vi "Main - Process - Protected.vi"(8 "error in (no error)":errorcluster) -> (0 "error out":errorcluster)   [LabVIEW 2011]
doc: "This is a basic Queue Driven Message Handler VI. Most advanced LabVIEW programmers who code extensively in LabVIEW utilitze some variation of this VI. This is a starting point. Some key features need to be added. In particular a robust error handling routine should be added.\n\nAAL 9/09"
uses:
  Shared/QDMH Poly VIs/QDMH POLY Enqueue Strings.vi
  Shared/QDMH Poly VIs/QDMH POLY Enqueue String.vi
panel:
  out "Recent Cases":string
  out "Message Display":string
  in  "Cancel":bool
  in  "OK":bool
  # "Run this VI and run Main - Interrupt Process.vi.  When you press the Interrupt Process button, the interruption is controlled and only happens between Process 3 and Process 1.  Notice how the messages are queued at the same time in the Timeout case in this VI.\nAlso, consider writting a more intelligent block of code to intercept the messages coming in."
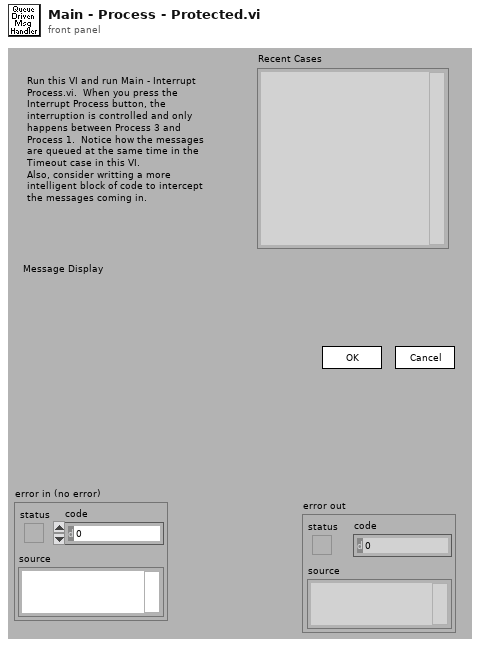
[diagram p1: front panel]
types:
  T1 = cluster{"Operator Name":string, "Current VI's Path":path, "Current VI's  Directory":path, "Queue Names":string[], "# VIs Launched":i32}
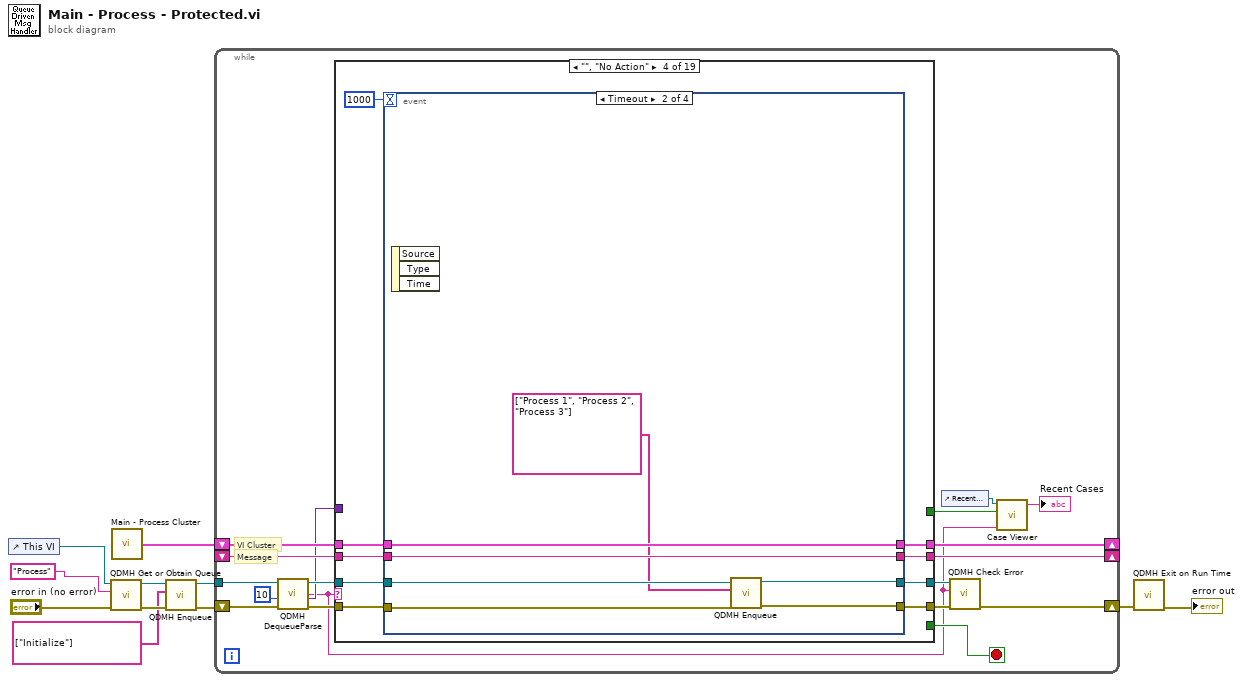
[diagram p0: block diagram]
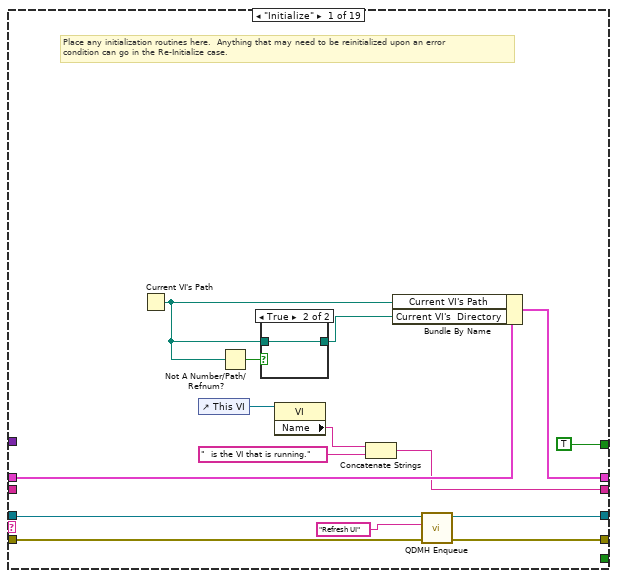
[diagram p2: hidden frame]
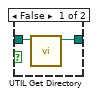
[diagram p3: hidden frame]
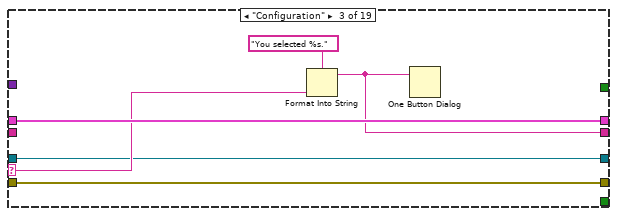
[diagram p5: hidden frame]
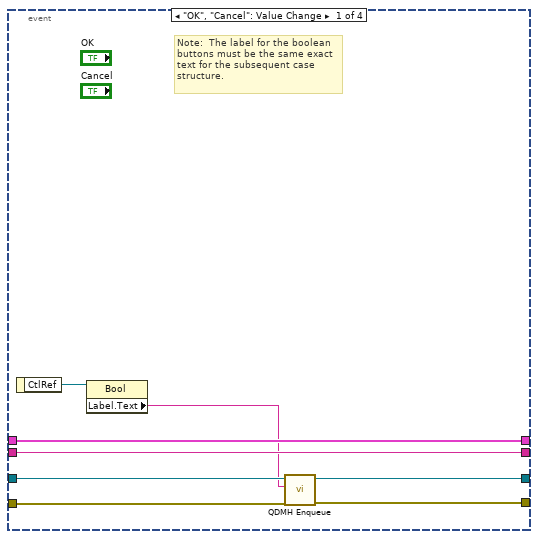
[diagram p6: hidden frame]
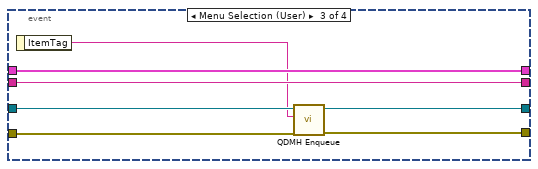
[diagram p7: hidden frame]
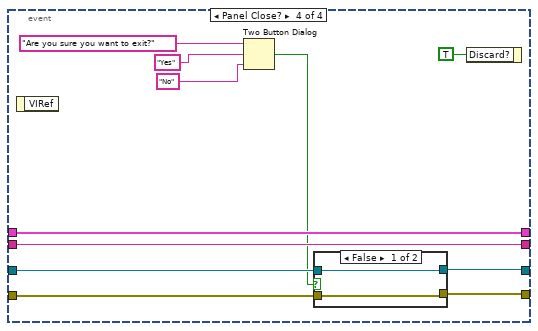
[diagram p8: hidden frame]
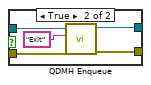
[diagram p9: hidden frame]
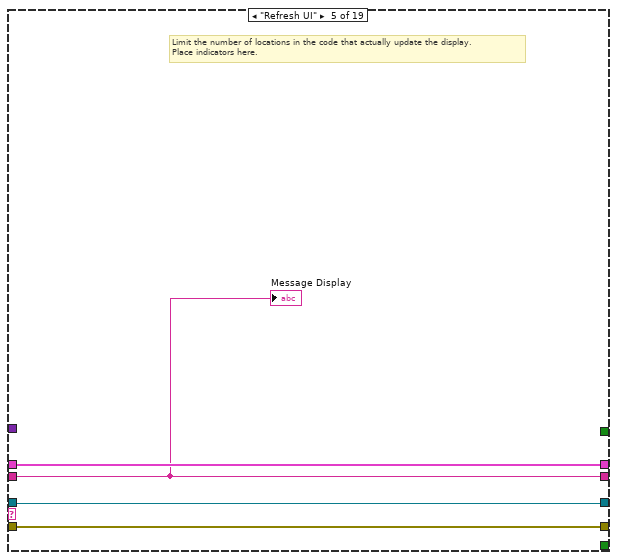
[diagram p10: hidden frame]
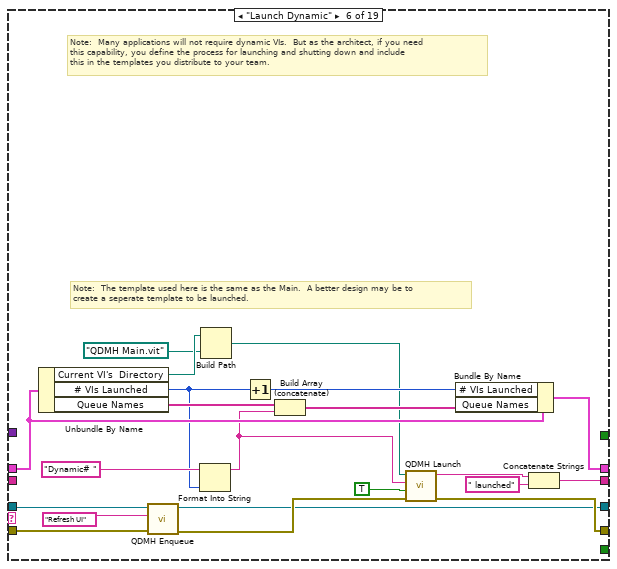
[diagram p11: hidden frame]
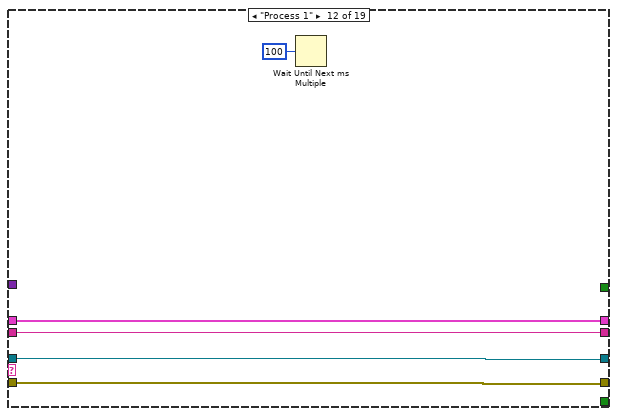
[diagram p17: hidden frame]
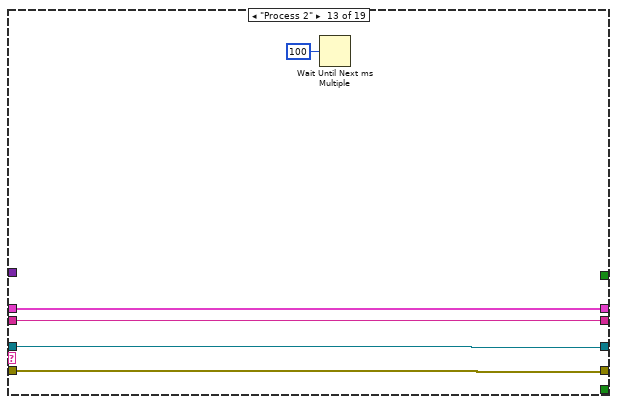
[diagram p18: hidden frame]
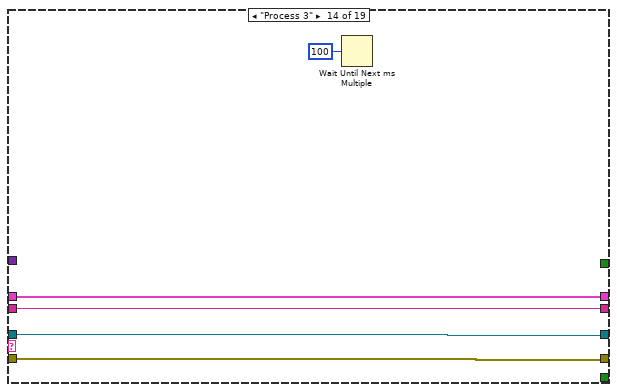
[diagram p19: hidden frame]
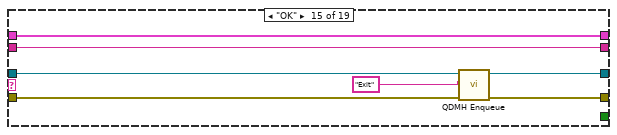
[diagram p20: hidden frame]
diagram:
  n1 = control-ref of="This VI"() -> (w5:refnum<vi>)
  n2 = call "QDMH Get or Obtain Queue.vi"("error in (no error)"="error in (no error)", "Queue Name"="Process", "VI Refnum"=w5) -> ("error out"=w8:errorcluster, "queue out"=w9:refnum<queue>)  [unwired: 7 out]
  n3 = call "Main - Process Cluster.vi"() -> ("Cluster"=w11:T1)
  n4 = call-poly "QDMH Enqueue.vi"("error in (no error)"=w8, "States"=string[] ["Initialize"], "queue"=w9) -> ("error out"=w6:errorcluster, "queue out"=w7:refnum<queue>)  [unwired: 7 out]
  n5 = while {
    tunnel: w7 -> [w24]
    shift-left: w11 -> [w25]
    shift-right: [w26] -> _
    shift-left: _ -> [w27]
    shift-right: [w28] -> _
    shift-right: [w18] -> w4
    shift-left: w6 -> [w20]
    stop <- w29 stop-if-true
    # "VI Cluster"
    # "Message"
    n6 = call "QDMH DequeueParse.vi"("error in (no error)"=w20, "Timeout"=10 ("ms timeout (-1)"), "queue"=w24) -> ("error out"=w21:errorcluster, "Variant Data"=w16:variant, "State"=w12:string, "queue out"=w22:refnum<queue>)  [unwired: 5 out]
    n7 = case shown="\"\", \"No Action\"" w12 {
      selector: w12 -> [_ _ w54 _ _ _ _ _ _ _ _ _ _ _ _ _ _ w193 _]
      tunnel: w22 -> [w40 w48 w53 w66 w108 w127 w132 w136 w140 w144 w148 w154 w159 w164 w173 w175 w187 w190 w203]
      tunnel: [_ _ _ _ _ _ _ _ _ _ _ _ _ _ _ _ _ _ TRUE] -> w29
      tunnel: [w38 w51 w55 w59 w109 w128 w135 w139 w143 w147 w151 w156 w161 w166 w172 w177 w189 w196 w205] -> w28
      tunnel: w27 -> [_ w51 _ w60 w109 _ w135 w139 w143 w147 w151 w156 w161 w166 w172 w177 w189 w196 w205]
      tunnel: [w43 w50 w57 w61 w110 w124 w134 w138 w142 w146 w150 w155 w160 w165 w171 w176 w188 w195 w200] -> w26
      tunnel: w25 -> [w44 w50 w57 w62 w110 w125 w134 w138 w142 w146 w150 w155 w160 w165 w171 w176 w188 w195 w200]
      tunnel: w21 -> [w42 w49 w52 w65 w107 w118 w133 w137 w141 w145 w149 w153 w158 w163 w170 w174 _ w192 w202]
      tunnel: [w41 w49 w52 w64 w107 w117 w133 w137 w141 w145 w149 w153 w158 w163 w169 w174 w186 w192 w197] -> w19
      tunnel: [w33 w48 w53 w58 w108 w114 w132 w136 w140 w144 w148 w154 w159 w164 w167 w175 w185 w190 refnum<queue> refnum ("queue out")] -> w17
      tunnel: w16 -> [_ _ _ _ _ _ _ _ _ _ _ _ _ _ _ _ w183 _ _]
      tunnel: [TRUE _ _ _ _ _ _ _ _ _ _ _ _ _ _ _ _ _ _] -> w14
      frame "Initialize" {
        # "Place any initialization routines here.  Anything that may need to be reinitialized upon an error\ncondition can go in the Re-Initialize case."
        n8 = Current VI's Path() -> (path=w31:path)
        n9 = control-ref of="This VI"() -> (w37:refnum<vi>)
        n10 = Not A Number/Path/Refnum?(number/path/refnum=w31) -> (NaN/Path/Refnum?=w32:bool)
        n11 = case shown="True" w32 {
          tunnel: w31 -> [w46 w47]
          tunnel: [w45 w47] -> w35
          frame False {
            n12 = call "UTIL Get Directory.vi"("Path In"=w46) -> ("Directory Out"=w45:path)  [unwired: 1 in, 9 out]
          }
          frame True {
          }
        }
        n13 = property class="VI"(reference=w37) -> ("Name"=w36:string)  [unwired: 1 in, 2 out]
        n14 = Concatenate Strings(w36, "  is the VI that is running." ("string")) -> (w38:string)
        n15 = Bundle By Name(cluster=w44, "Current VI's Path"=w31, "Current VI's  Directory"=w35) -> (w43:T1)
        n16 = call-poly "QDMH Enqueue.vi"("error in (no error)"=w42, "State"="Refresh UI" ("New State"), "queue"=w40) -> ("error out"=w41:errorcluster, "queue out"=w33:refnum<queue>)  [unwired: 7 out]
      }
      frame "Re-Initialize" {
        # "This case includes initialization functionality that may need to run again during the course of the VI"
      }
      frame "Configuration" {
        n17 = Format Into String(format string="You selected %s." ("Format String"), w54) -> (resulting string=w55:string)  [unwired: 2 in, 1 out]
        n18 = One Button Dialog(message=w55) -> ()  [unwired: 2 out]
      }
      frame "", "No Action" {
        n19 = event shown="[1] Timeout" {
          selector: _ -> [_ _ _ _]
          dyn-events: _ -> [_ _ _ _]
          timeout: 1000 -> [_ _ _ _]
          tunnel: w66 -> [w73 w79 w88 w95]
          tunnel: [w72 w76 w86 w92] -> w64
          tunnel: w65 -> [w71 w78 w87 w94]
          tunnel: w62 -> [w70 w81 w85 w99]
          tunnel: [w70 w81 w85 w99] -> w61
          tunnel: w60 -> [w69 w80 w84 w98]
          tunnel: [w69 w80 w84 w98] -> w59
          tunnel: [w67 w77 w82 w93] -> w58
          event "OK", "Cancel": Value Change {
            # "Note:  The label for the boolean buttons must be the same exact text for the subsequent case structure."
            n20 = event-data() -> ("CtlRef"=w74:refnum<vi>)  [unwired: 1 out]
            n21 = property class="Bool"(reference=w74) -> ("Label.Text"=w68:string)  [unwired: 1 in, 2 out]
            n22 = call-poly "QDMH Enqueue.vi"("error in (no error)"=w71, "State"=w68, "queue"=w73) -> ("error out"=w72:errorcluster, "queue out"=w67:refnum<queue>)  [unwired: 7 out]
          }
          event Timeout {
            n23 = event-data() -> ()  [unwired: 4 out]
            n24 = call-poly "QDMH Enqueue.vi"("error in (no error)"=w78, "States"=string[] ["Process 1", "Process 2", "Process 3"], "queue"=w79) -> ("error out"=w76:errorcluster, "queue out"=w77:refnum<queue>)  [unwired: 7 out]
          }
          event Menu Selection (User) {
            n25 = event-data() -> ("ItemTag"=w83:string)  [unwired: 1 out]
            n26 = call-poly "QDMH Enqueue.vi"("error in (no error)"=w87, "State"=w83, "queue"=w88) -> ("error out"=w86:errorcluster, "queue out"=w82:refnum<queue>)  [unwired: 7 out]
          }
          event Panel Close? {
            n27 = event-data() -> ()  [unwired: 2 out]
            n28 = Two Button Dialog(message="Are you sure you want to exit?", 1:"No" ("T button name (\"OK\")"), 2:"Yes" ("F button name (\"Cancel\")")) -> (T button?=w89:bool)
            n29 = case shown="False" w89 {
              tunnel: w95 -> [w101 w106]
              tunnel: w94 -> [w100 w105]
              tunnel: [w101 w104] -> w93
              tunnel: [w100 w103] -> w92
              frame False {
              }
              frame True {
                n30 = call-poly "QDMH Enqueue.vi"("error in (no error)"=w105, "State"="Exit", "queue"=w106) -> ("error out"=w103:errorcluster, "queue out"=w104:refnum<queue>)  [unwired: 7 out]
              }
            }
            n31 = event-data("Discard?"=TRUE) -> ()  [unwired: 1 in, 1 out]
          }
        }
      }
      frame "Refresh UI" {
        # "Limit the number of locations in the code that actually update the display.\nPlace indicators here."
        "Message Display" <- w109
      }
      frame "Launch Dynamic" {
        # "Note:  The template used here is the same as the Main.  A better design may be to\ncreate a seperate template to be launched."
        # "Note:  Many applications will not require dynamic VIs.  But as the architect, if you need\nthis capability, you define the process for launching and shutting down and include\nthis in the templates you distribute to your team."
        n32 = Unbundle By Name(w125) -> ("Current VI's  Directory"=w113:path, "# VIs Launched"=w121:i32, "Queue Names"=w123:string[])
        n33 = call-poly "QDMH Enqueue.vi"("error in (no error)"=w118, "State"="Refresh UI" ("New State"), "queue"=w127) -> ("error out"=w116:errorcluster, "queue out"=w114:refnum<queue>)  [unwired: 7 out]
        n34 = Format Into String(initial string="Dynamic# ", w121) -> (resulting string=w119:string)  [unwired: 2 in, 1 out]
        n35 = Build Path(base path=w113, name or relative path=path "QDMH Main.vit" ("vi path")) -> (appended path=w111:path)
        n36 = Increment(x=w121) -> (x+1=w120:i32)
        n37 = Build Array (concatenate)(w123, w119) -> (w122:string[])
        n38 = call "QDMH Launch.vi"("error in (no error)"=w116, "Front Panel Window (Open)"=TRUE ("Front Panel Window:Open"), "Queue Name"=w119, "VI Path"=w111) -> ("error out"=w117:errorcluster, "Launched VI Name"=w130:string)  [unwired: 6 out]
        n39 = Bundle By Name(cluster=w125, "# VIs Launched"=w120, "Queue Names"=w122) -> (w124:T1)
        n40 = Concatenate Strings(w130, " launched" ("string")) -> (w128:string)
      }
      frame "Shutdown Dynamic" {
      }
      frame "Send Message to Dynamic" {
      }
      frame "Receive Message From Dynamic" {
      }
      frame "<duplicate me for new states >" {
        # "Duplicate this state for any additional states that you add."
      }
      frame "Interrupt Process" {
        # "Duplicate this state for any additional states that you add."
      }
      frame "Process 1" {
        n41 = Wait Until Next ms Multiple(millisecond multiple=u32 100) -> ()  [unwired: 1 out]
      }
      frame "Process 2" {
        n42 = Wait Until Next ms Multiple(millisecond multiple=u32 100) -> ()  [unwired: 1 out]
      }
      frame "Process 3" {
        n43 = Wait Until Next ms Multiple(millisecond multiple=u32 100) -> ()  [unwired: 1 out]
      }
      frame "OK" {
        n44 = call-poly "QDMH Enqueue.vi"("error in (no error)"=w170, "State"="Exit" ("New State"), "queue"=w173) -> ("error out"=w169:errorcluster, "queue out"=w167:refnum<queue>)  [unwired: 7 out]
      }
      frame "Cancel" {
      }
      frame "Error" {
        # "This codes simply displays an error dialog that will allow the user\nto continue code execution or Exit.  More error correction code\ncould be included.  This will be explored in the error system exercise."
        n45 = Variant To Data(type=cluster{"Case":string, "error":errorcluster} {"Case"="", "error"={"status"=FALSE, "code"=0, "source"=""}} ("QDSM Element"), Variant=w183) -> (data=w182:cluster{"Case":string, "error":errorcluster})  [unwired: 1 in, 1 out]
        n46 = Unbundle By Name(w182) -> ("Case"=w181:string, "error"=w180:errorcluster)
        n47 = call "QDMH Error Dialog.vi"("error"=w180, "Case Error Occured"=w181) -> ("error out (no error)"=w178:errorcluster, "Case to Execute"=w179:string)  [unwired: 8 out]
        n48 = call-poly "QDMH Enqueue.vi"("error in (no error)"=w178, "State"=w179, "queue"=w187) -> ("error out"=w186:errorcluster, "queue out"=w185:refnum<queue>)  [unwired: 7 out]
      }
      frame "Developer Error", Default {
        # "Many eschew the use of string based state machines because of the propensity for\ntypos, prefering instead to use enums.  This case eliminates that concern.\nPerhaps modify to exit the VI."
        n49 = Format Into String(format string="Developer Error: The requested state \"%s\" does not exist." ("message"), w193) -> (resulting string=w191:string)  [unwired: 2 in, 1 out]
        n50 = One Button Dialog(message=w191) -> ()  [unwired: 2 out]
      }
      frame "Exit" {
        # "Note:  The release queue function has the force destroy option set to true."
        # "Place any critical clean up routines here."
        n51 = Unbundle By Name(w200) -> ("Queue Names"=w198:string[])
        n52 = Release Queue(queue=w203, force destroy? (F)=TRUE, error in (no error)=w202) -> (error out=w197:errorcluster)  [unwired: 2 out]
        n53 = for {
          tunnel: w198 -> [w210] mode=indexing
          n54 = Obtain Queue(name (unnamed)=w210, element data type=cluster{"State":string, "Variant Data":variant} {"State"="", "Variant Data"=variant} ("QDSM Element")) -> (queue out=w209:refnum<queue>)  [unwired: 3 in, 2 out]
          n55 = call-poly "QDMH Enqueue.vi"("State"="Exit" ("element"), "queue"=w209) -> ()  [unwired: 1 in, 9 out]
        }
        n56 = local write "Message Display"("") -> ()
      }
    }
    n57 = control-ref of="Recent Cases"() -> (w13:refnum<vi>)
    n58 = call "QDMH Check Error.vi"("error in (no error)"=w19, "Case"=w12, "queue"=w17) -> ("error out"=w18:errorcluster)  [unwired: 1 in, 7 out]
    n59 = call "Case Viewer.vi"("Case"=w12, "Flush?"=w14, "Str Refnum"=w13) -> ("Recent Cases"=→"Recent Cases":string)  [unwired: 8 in]
  }
  n60 = call "QDMH Exit on Run Time.vi"("error in (no error)"=w4) -> ("error out"=→"error out":errorcluster)  [unwired: 10 in]
